vi "写文件.vi"   [LabVIEW 2021]
doc: "本VI是为《我和LabVIEW》一书编写的示例。\n关于本书的介绍请参考网页：\nhttp://ruanqizhen.spaces.live.com/blog/cns!5852D4F797C53FB6!4310.entry"
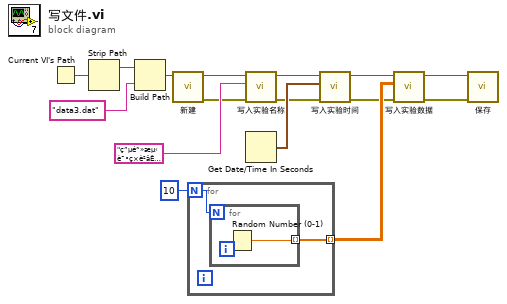
[diagram p0: block diagram]
diagram:
  n1 = Current VI's Path() -> (path=w16:path)
  n2 = Strip Path(path=w16) -> (stripped path=w15:path)  [unwired: 1 out]
  n3 = Build Path(base path=w15, name or relative path="data3.dat" ("名称或相对路径")) -> (appended path=w12:path)
  n4 = call "新建.vi"("路径"=w12) -> ("error out"=w5:errorcluster, "数据文件.lvclass"=w11:refnum<class "数据文件.lvclass">)  [unwired: 9 in]
  n5 = for {
    N: 10 -> [w18]
    tunnel: [w17] -> w8 mode=indexing
    n6 = for {
      N: w18 -> [_]
      tunnel: [w19] -> w17 mode=indexing
      n7 = Random Number (0-1)() -> (number: 0 to 1=w19:dbl)
    }
  }
  n8 = call-dynamic "写入实验名称.vi"("error in (no error)"=w5, "实验名称"="ç”µé˜»æµ‹è¯•ç×è²âÊÔ", "数据文件.lvclass"=w11) -> ("error out"=w4:errorcluster, "数据文件.lvclass"=w6:refnum<class "数据文件.lvclass">)  [unwired: 7 in]
  n9 = Get Date/Time In Seconds() -> (seconds since 1Jan1904=w9:timestamp)
  n10 = call-dynamic "写入实验时间.vi"("error in (no error)"=w4, "实验时间"=w9, "数据文件.lvclass"=w6) -> ("error out"=w3:errorcluster, "数据文件.lvclass"=w7:refnum<class "数据文件.lvclass">)  [unwired: 7 in]
  n11 = call-dynamic "写入实验数据.vi"("error in (no error)"=w3, "实验数据"=w8, "数据文件.lvclass"=w7) -> ("error out"=w1:errorcluster, "数据文件.lvclass"=w2:refnum<class "数据文件.lvclass">)  [unwired: 7 in]
  n12 = call-dynamic "保存.vi"("error in (no error)"=w1, "数据文件.lvclass"=w2) -> ()  [unwired: 8 in, 2 out]
